vi "Close.vi"(8 "error in (no error)":errorcluster, 10 "Internal?":bool, 11 "Lauda  Settings":T1) -> (0 "error out":errorcluster, 3 "Lauda Settings":T1)   [LabVIEW 2018, in "Lauda TCU.lvlib"]
uses:
  Lauda TCU.lvlib
  Lauda Settings.ctl
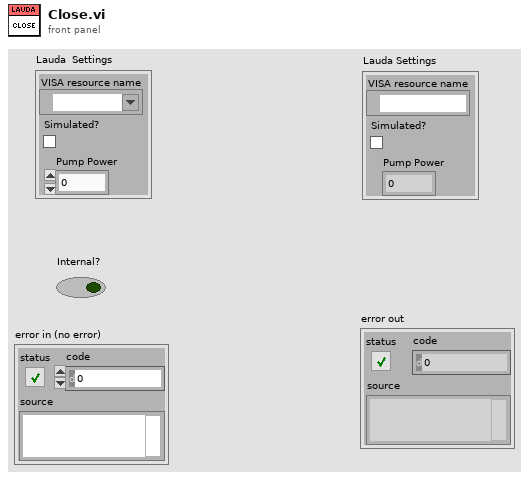
[diagram p1: front panel]
types:
  T1 = typedef "Lauda TCU.lvlib/Lauda Settings.ctl" = cluster{"VISA resource name":refnum<visa-resource-name>, "Simulated?":bool, "Pump Power":i32}
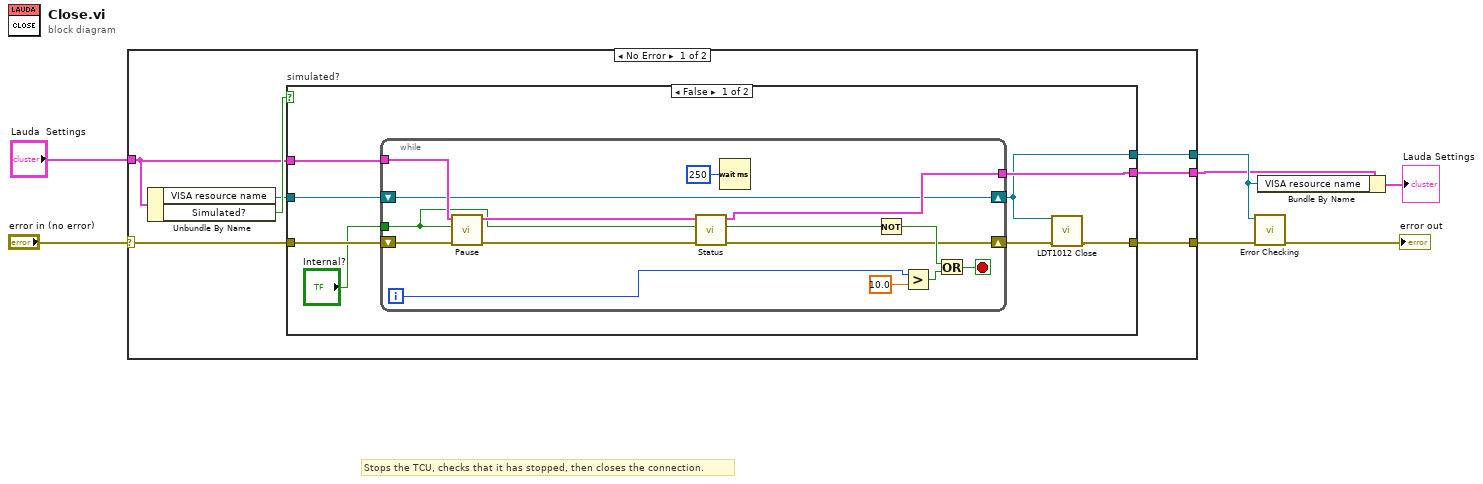
[diagram p0: block diagram]
diagram:
  # "Stops the TCU, checks that it has stopped, then closes the connection."
  n1 = case shown="No Error" "error in (no error)" {
    selector: "error in (no error)" -> [w12 w43]
    tunnel: [w13 w43] -> w6
    tunnel: "Lauda  Settings" -> [w9 w41]
    tunnel: [w10 w42] -> w4
    tunnel: [w8 w41] -> w3
    frame No Error {
      n2 = Unbundle By Name(w9) -> ("VISA resource name"=w11:refnum<visa-resource-name>, "Simulated?"=w14:bool)
      n3 = case "simulated?" shown="False" w14 {
        tunnel: [w16 w40] -> w13
        tunnel: w11 -> [w21 w39]
        tunnel: w12 -> [w22 w40]
        tunnel: [w18 w39] -> w10
        tunnel: w9 -> [w20 w38]
        tunnel: [w19 w38] -> w8
        frame False {
          n4 = while {
            shift-right: [w25] -> w17
            shift-left: w22 -> [w35]
            shift-right: [w26] -> w18
            shift-left: w21 -> [w26]
            tunnel: w20 -> [w34]
            tunnel: [w36] -> w19
            tunnel: "Internal?" -> [w23]
            i -> [w30]
            stop <- w27 stop-if-true
            n5 = call "Pause.vi"("error in (no error)"=w35, "Internal?"=w23, "Huber Settings"=w34) -> ("error out"=w24:errorcluster, "Huber Settings"=w33:T1)  [unwired: 7 in]
            n6 = call "Status.vi"("error in (no error)"=w24, "Internal?"=w23, "Lauda Settings"=w33) -> ("error out"=w25:errorcluster, "Running"=w37:bool, "Lauda Settings"=w36:T1)  [unwired: 2 in, 4 out]
            n7 = Wait (ms)(milliseconds to wait=u32 250) -> ()  [unwired: 1 out]
            n8 = Not(x=w37) -> (.not. x?=w28:bool)
            n9 = Greater?(x=w30, y=10.0) -> (0:w32:bool)
            n10 = Or(x=w28, y=w32) -> (x .or. y?=w27:bool)
          }
          n11 = call "LDT1012 Close.vi"("error in (no error)"=w17, "VISA session"=w18) -> ("error out"=w16:errorcluster)  [unwired: 9 in]
        }
        frame True {
        }
      }
    }
    frame Error {
      n12 = Unbundle By Name(w41) -> ("VISA resource name"=w42:refnum<visa-resource-name>)
    }
  }
  n13 = call "Error Checking.vi"("error in (no error)"=w6, "VISA resource name"=w4) -> ("error out"=→"error out":errorcluster)  [unwired: 7 in, 2 out]
  n14 = Bundle By Name(cluster=w3, "VISA resource name"=w4) -> (→"Lauda Settings":T1)
